vi "Host-Top-Level.vi"() -> ()   [LabVIEW 2016]
uses:
  <vilib>/rvi/interface/RandomDataEmulation/nirviRandomDataOpen.vi
  <vilib>/rvi/interface/common/niFpgaCacheSessionInfoDynamic.vi
  <vilib>/Utility/error.llb/Error Cluster From Error Code.vi
  <vilib>/rvi/errors/niLvFpgaAdjustHostInterfaceError.vi
  <vilib>/FPGAPlugInAG/Dynamic/niLvFpga_Close_Dynamic.vi
  <vilib>/rvi/interface/nirviOpenFPGA/nirviOpenFPGA.xnode
  Fpga-Top-Level.vi
  <vilib>/rvi/interface/nirviMethod/nirviMethod.xnode
  <vilib>/rvi/interface/nirviCloseFPGA/nirviCloseFPGA.xnode
  <vilib>/FPGAPlugInAG/Dynamic/niLvFpga_ReadFifo_Dynamic.vi
  <vilib>/rvi/errors/niLvFpgaMergeErrorWithErrorCode.vi
panel:
  in  "Clear":bool
  out "Data":u32[](array[numeric])
  in  "Read":bool
  in  "error in":errorcluster
  out "Message":string="ERROR!"
  in  "Exit":bool
  in  "Start":bool
  in  "file path (use dialog)":path
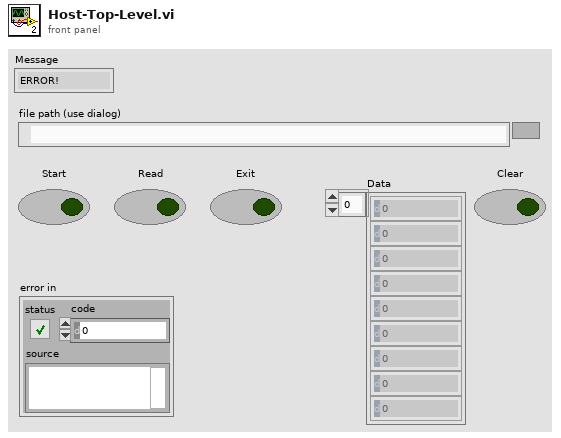
[diagram p1: front panel]
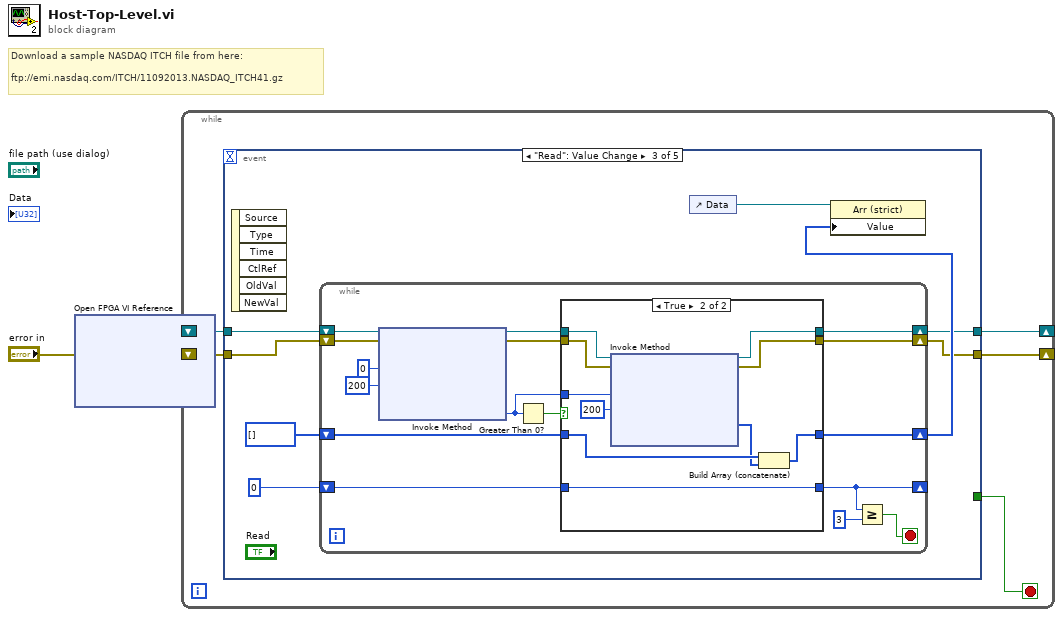
[diagram p0: block diagram]
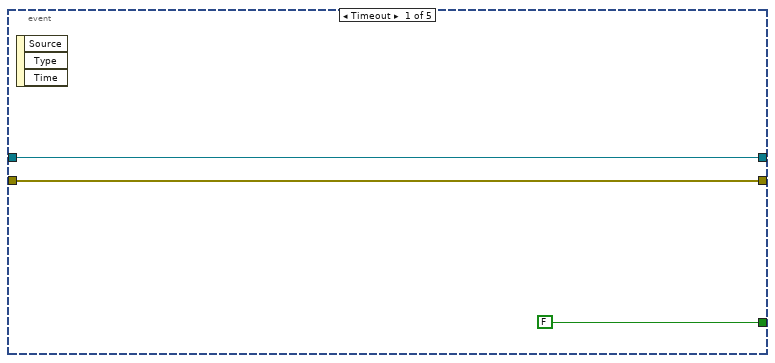
[diagram p2: hidden frame]
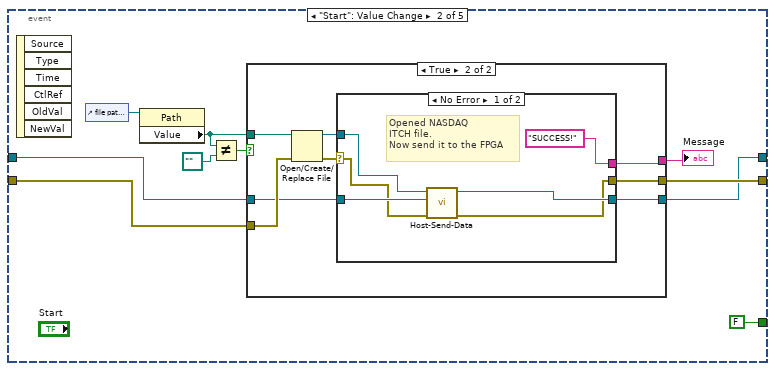
[diagram p3: hidden frame]
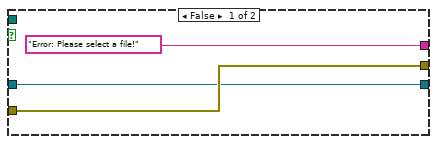
[diagram p4: hidden frame]
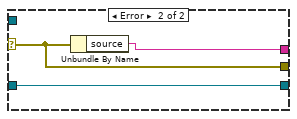
[diagram p5: hidden frame]
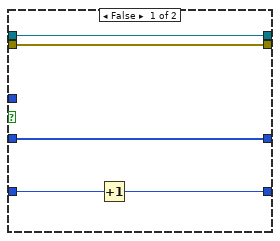
[diagram p6: hidden frame]
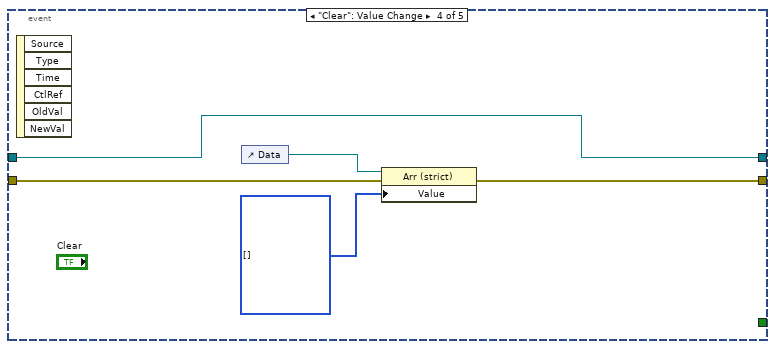
[diagram p7: hidden frame]
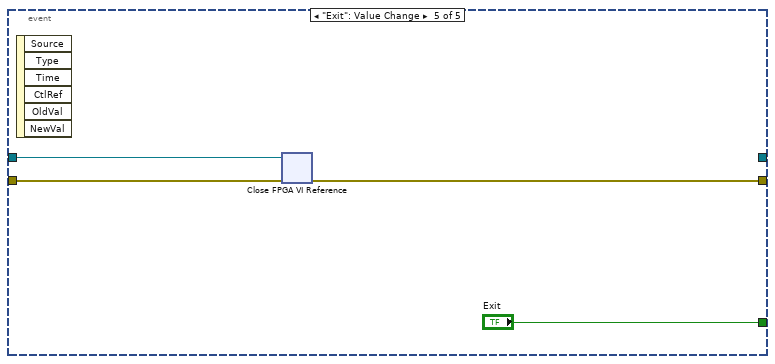
[diagram p8: hidden frame]
diagram:
  # "Download a sample NASDAQ ITCH file from here:\n\nftp://emi.nasdaq.com/ITCH/11092013.NASDAQ_ITCH41.gz"
  n1 = xnode "Open FPGA VI Reference"("error in"="error in") -> ("FPGA VI Reference Out"=w1:refnum<k20>, "error out"=w2:errorcluster)  [unwired: 1 in]
  n2 = while {
    shift-right: [w6] -> _
    shift-left: w2 -> [w7]
    shift-right: [w5] -> _
    shift-left: w1 -> [w4]
    stop <- w8 stop-if-true
    n3 = event shown="[2] \"Read\": Value Change" {
      selector: _ -> [_ _ _ _ _]
      dyn-events: _ -> [_ _ _ _ _]
      timeout: _ -> [_ _ _ _ _]
      tunnel: [FALSE ("Exit") FALSE ("Exit") _ _ "Exit"] -> w8
      tunnel: w7 -> [w10 w15 w46 w83 w88]
      tunnel: [w10 w13 w42 w82 w87] -> w6
      tunnel: [w9 w12 w43 w81 _] -> w5
      tunnel: w4 -> [w9 w14 w48 w81 w86]
      event Timeout {
        n4 = event-data() -> ()  [unwired: 1 in, 3 out]
      }
      event "Start": Value Change {
        n5 = event-data() -> ()  [unwired: 1 in, 6 out]
        n6 = control-ref of="file path (use dialog)"() -> (w20:refnum<vi>)
        n7 = property class="Path"(reference=w20) -> ("Value"=w19:path)  [unwired: 1 in, 2 out]
        n8 = Not Equal?(x=w19, y=path "" ("Value")) -> (x != y?=w17:bool)
        n9 = case shown="True" w17 {
          tunnel: w19 -> [_ w32]
          tunnel: ["Error: Please select a file!" w29] -> w16
          tunnel: w15 -> [w23 w31]
          tunnel: w14 -> [w22 w28]
          tunnel: [w23 w27] -> w13
          tunnel: [w22 w26] -> w12
          frame False {
          }
          frame True {
            n10 = Open/Create/Replace File(file path (use dialog)=w32, error in=w31) -> (refnum out=w25:refnum<file>, error out=w30:errorcluster)  [unwired: 4 in, 1 out]
            n11 = case shown="No Error" w30 {
              selector: w30 -> [w35 w39]
              tunnel: ["SUCCESS!" w41] -> w29
              tunnel: w28 -> [w37 w40]
              tunnel: [w33 w39] -> w27
              tunnel: [w36 w40] -> w26
              tunnel: w25 -> [w34 _]
              frame No Error {
                # "Opened NASDAQ\nITCH file.\nNow send it to the FPGA"
                n12 = call "Host-Send-Data.vi"("error in\n(no error)"=w35, "FPGA VI Reference In"=w37, "Byte Stream\nFile in"=w34) -> ("error out"=w33:errorcluster, "FPGA VI Reference Out"=w36:refnum<k20>)  [unwired: 7 in]
              }
              frame Error {
                n13 = Unbundle By Name(w39) -> ("source"=w41:string)
              }
            }
          }
        }
        "Message" <- w16
      }
      event "Read": Value Change {
        n14 = event-data() -> ()  [unwired: 1 in, 6 out]
        n15 = while {
          shift-right: [w54] -> w44
          shift-left: u32[] [] ("Data 2") -> [w55]
          shift-right: [w57] -> w43
          shift-left: w48 -> [w65]
          shift-right: [w56] -> w42
          shift-left: w46 -> [w58]
          shift-right: [w52] -> _
          shift-left: 0 -> [w53]
          stop <- w50 stop-if-true
          n16 = xnode "Invoke Method"("FPGA VI Reference In"=w65, "error in"=w58, "Number of Elements"=u32 0, "Timeout (ms)"=200) -> ("FPGA VI Reference Out"=w60:refnum<k20>, "error out"=w59:errorcluster, "Elements Remaining"=w61:u32)  [unwired: 1 out]
          n17 = Greater Than 0?(x=w61) -> (x > 0?=w62:bool)
          n18 = case shown="True" w62 {
            tunnel: w61 -> [_ w80]
            tunnel: w60 -> [w70 w78]
            tunnel: w59 -> [w69 w77]
            tunnel: [w70 w76] -> w57
            tunnel: [w69 w75] -> w56
            tunnel: w55 -> [w68 w74]
            tunnel: [w68 w72] -> w54
            tunnel: [w66 w71] -> w52
            tunnel: w53 -> [w67 w71]
            frame False {
              n19 = Increment(x=w67) -> (x+1=w66:i32)
            }
            frame True {
              n20 = xnode "Invoke Method"("FPGA VI Reference In"=w78, "error in"=w77, "Number of Elements"=w80, "Timeout (ms)"=200) -> ("FPGA VI Reference Out"=w76:refnum<k20>, "error out"=w75:errorcluster, "Data"=w73:u32[])  [unwired: 1 out]
              n21 = Build Array (concatenate)(w74, w73) -> (w72:u32[])
            }
          }
          n22 = Greater Or Equal?(x=w52, y=3) -> (x >= y?=w50:bool)
        }
        n23 = control-ref of="Data"() -> (w49:refnum<vi>)
        n24 = property class="Arr (strict)"(reference=w49, "Value"=w44) -> ()  [unwired: 1 in, 2 out]
      }
      event "Clear": Value Change {
        n25 = event-data() -> ()  [unwired: 1 in, 6 out]
        n26 = control-ref of="Data"() -> (w84:refnum<vi>)
        n27 = property class="Arr (strict)"(reference=w84, error in=w83, "Value"=u32[] []) -> (error out=w82:errorcluster)  [unwired: 1 out]
      }
      event "Exit": Value Change {
        n28 = event-data() -> ()  [unwired: 1 in, 6 out]
        n29 = xnode "Close FPGA VI Reference"("FPGA VI Reference In"=w86, "error in"=w88) -> ("error out"=w87:errorcluster)
      }
    }
  }
